vi "CheckRunGolden.vi"() -> ()   [LabVIEW 2012]
uses:
  <vilib>/addons/database/Auxilliary.llb/DB Tools Cursor Type.ctl
  <vilib>/addons/database/Connection.llb/DB Tools Open Connec (Path).vi
  <vilib>/addons/database/Connection.llb/Conn Execute.vi
  <vilib>/addons/database/Recordset.llb/Rec Destroy - Connection.vi
  <vilib>/addons/database/Recordset.llb/Rec Fetch Recordset Data (R).vi
  <vilib>/addons/database/_DB Variant To Data/Database Variant To Data.xnode
  <vilib>/addons/database/NI_Database_API.lvlib
panel:
  out "error out":errorcluster
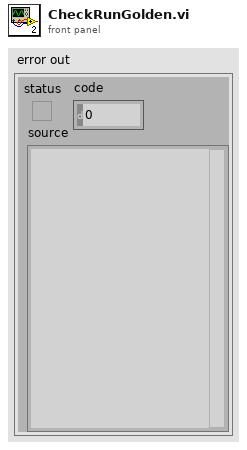
[diagram p1: front panel]
types:
  T1 = typedef "NI_Database_API.lvlib/DB Tools Cursor Type.ctl" = enum16{"forward-only", "keyset", "dynamic", "static"}
  T2 = typedef "NI_Database_API.lvlib/Conn ObjectReference.ctl" = refnum<k1>
  T3 = typedef "NI_Database_API.lvlib/Rec ObjectReference.ctl" = refnum<k1>
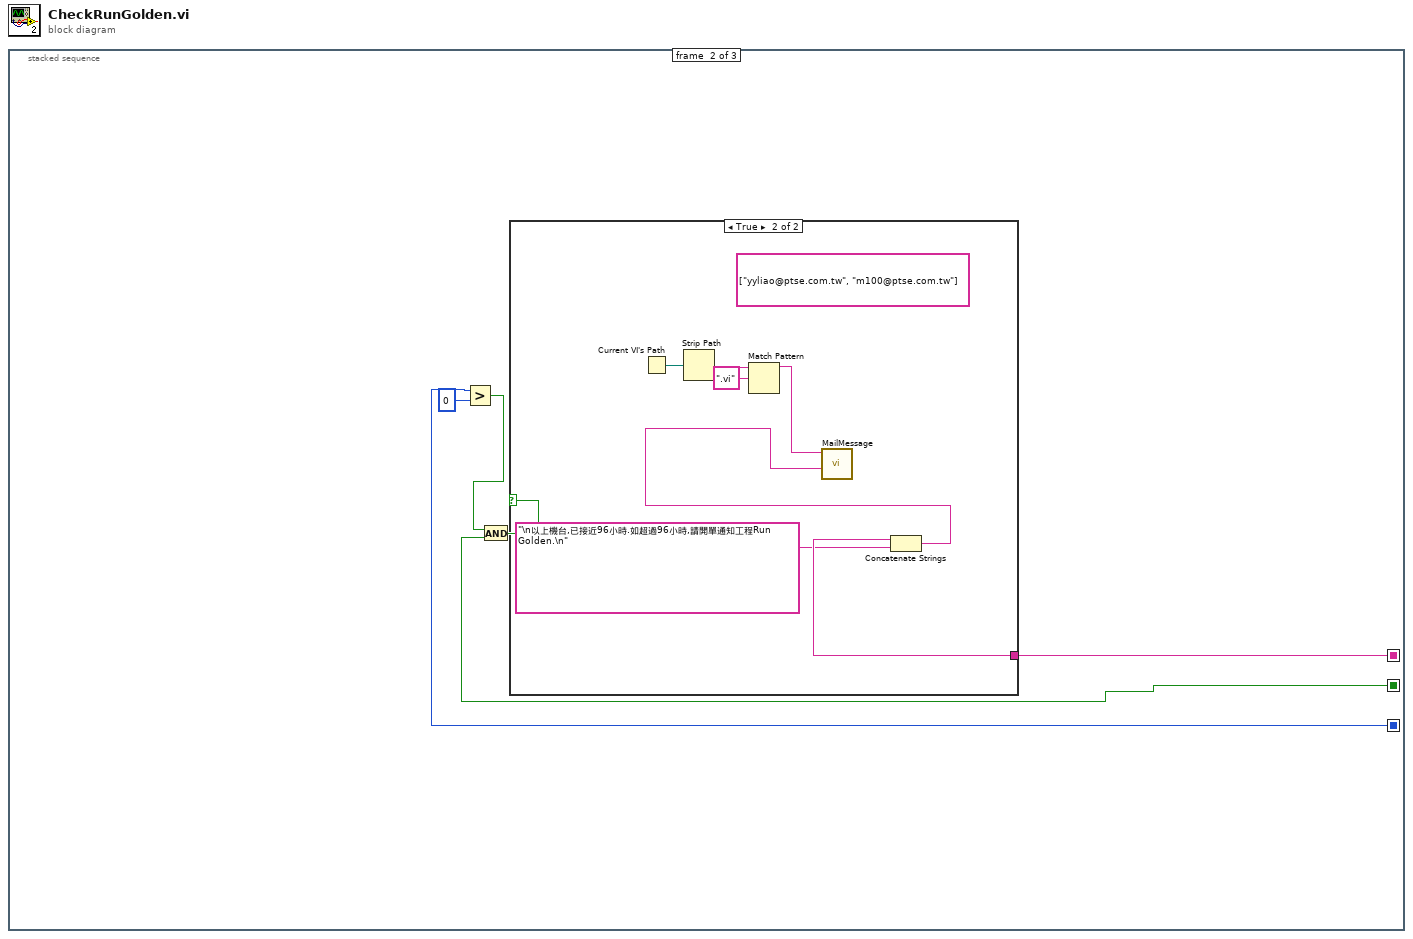
[diagram p0: block diagram]
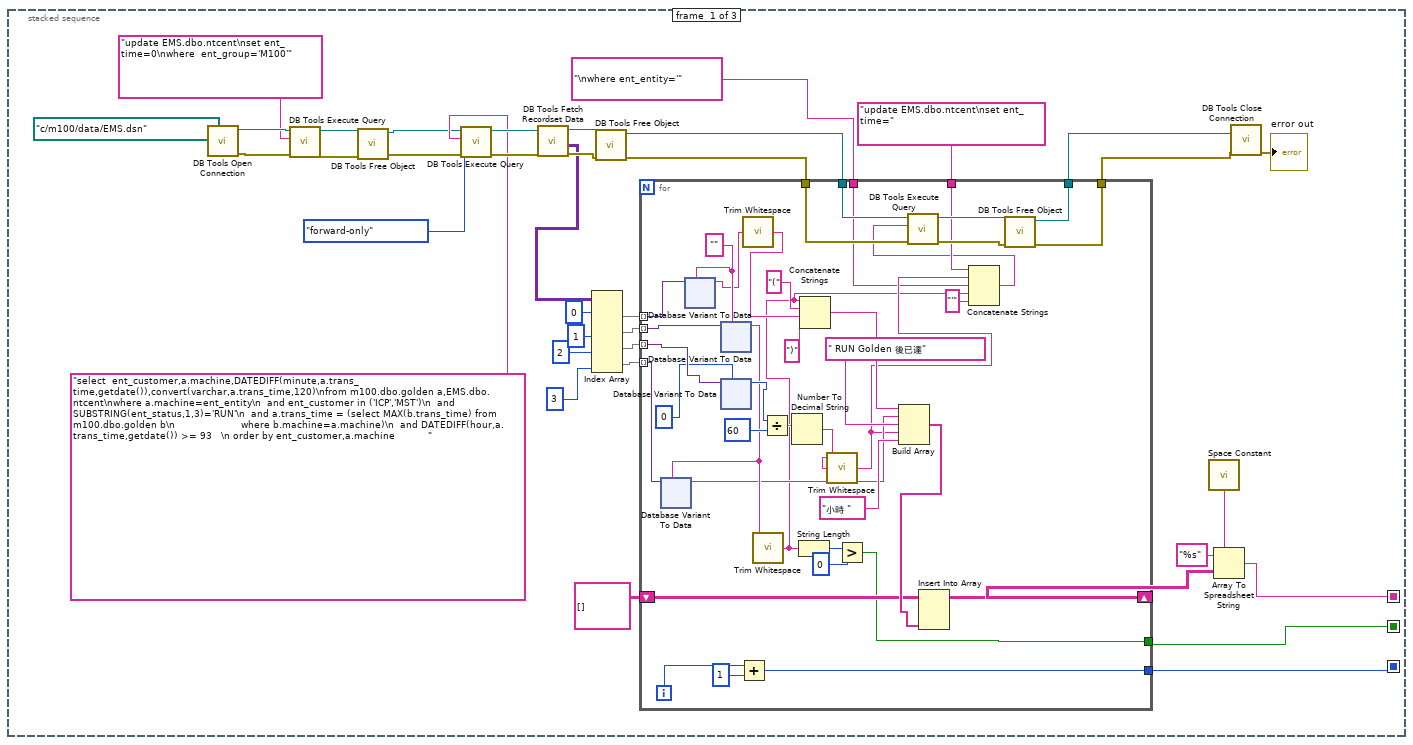
[diagram p2: hidden frame]
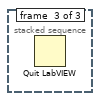
[diagram p4: hidden frame]
diagram:
  n1 = stacked-sequence {
    seq-local: [w24 _ _] -> [_ w211 _]
    seq-local: [w22 _ _] -> [_ w210 _]
    seq-local: [w21 _ _] -> [_ w206 _]
    frame #0 {
      n2 = call-poly <vilib>:"DB Tools Open Connection.vi"("connection information"=path "c:/m100/data/EMS.dsn") -> ("error out"=w2:errorcluster, "connection reference"=w8:T2)  [unwired: 7 in]
      n3 = call-poly <vilib>:"DB Tools Execute Query.vi"("error in (no error)"=w2, "SQL query"="update EMS.dbo.ntcent\nset ent_time=0\nwhere  ent_group='M100'", "connection reference"=w8) -> ("error out"=w3:errorcluster, "recordset reference"=w7:T3)  [unwired: 5 in]
      n4 = call-poly <vilib>:"DB Tools Free Object.vi"("error in (no error)"=w3, "recordset reference"=w7) -> ("error out"=w4:errorcluster, "connection reference"=w5:T2)  [unwired: 8 in]
      n5 = call-poly <vilib>:"DB Tools Execute Query.vi"("error in (no error)"=w4, "cursor type"=DB_Tools_Cursor_Type."forward-only", "SQL query"="select  ent_customer,a.machine,DATEDIFF(minute,a.trans_time,getdate()),convert(varchar,a.trans_time,120)\nfrom m100.dbo.golden a,EMS.dbo.ntcent\nwhere a.machine=ent_entity\n  and ent_customer in ('ICP','MST')\n  and SUBSTRING(ent_status,1,3)='RUN'\n  and a.trans_time = (select MAX(b.trans_time) from m100.dbo.golden b\n                      where b.machine=a.machine)\n  and DATEDIFF(hour,a.trans_time,getdate()) >= 93   \n order by ent_customer,a.machine           ", "connection reference"=w5) -> ("error out"=w35:errorcluster, "recordset reference"=w36:T3)  [unwired: 4 in]
      n6 = call-poly <vilib>:"DB Tools Fetch Recordset Data.vi"("error in (no error)"=w35, "recordset reference"=w36) -> ("error out"=w33:errorcluster, "recordset data"=w19:variant[][], "recordset reference out"=w34:T3)  [unwired: 3 in]
      n7 = Index Array(array=w19, index (col) #1=0 ("disabled index (col)"), index (col) #2=1 ("disabled index (col)"), index (col) #3=2 ("index (col)"), index (col) #4=3 ("index (col)")) -> (element #1=w17:variant[], element #2=w28:variant[], element #3=w27:variant[], element #4=w15:variant[])  [unwired: 4 in]
      n8 = call-poly <vilib>:"DB Tools Free Object.vi"("error in (no error)"=w33, "recordset reference"=w34) -> ("error out"=w12:errorcluster, "connection reference"=w14:T2)  [unwired: 8 in]
      n9 = for {
        tunnel: w28 -> [w77] mode=indexing
        tunnel: w27 -> [w76] mode=indexing
        shift-right: [w74] -> w25
        shift-left: string[][] [] -> [w73]
        tunnel: [w70] -> w22
        tunnel: [w67] -> w21
        tunnel: w17 -> [w59] mode=indexing
        tunnel: w15 -> [w53] mode=indexing
        tunnel: w14 -> [w49]
        tunnel: w12 -> [w48]
        tunnel: [w45] -> w13
        tunnel: [w44] -> w11
        tunnel: "update EMS.dbo.ntcent\nset ent_time=" -> [w43]
        tunnel: "\nwhere ent_entity='" ("string") -> [w41]
        i -> [w72]
        w58 = ""
        n10 = xnode "Database Variant To Data"("database variant"=w59, "type"=w58) -> ("data"=w55:string)  [unwired: 1 in, 1 out]
        n11 = xnode "Database Variant To Data"("database variant"=w77, "type"=w58) -> ("data"=w52:string)  [unwired: 1 in, 1 out]
        n12 = xnode "Database Variant To Data"("database variant"=w53, "type"=w52) -> ("data"=w50:string)  [unwired: 1 in, 1 out]
        n13 = xnode "Database Variant To Data"("database variant"=w76, "type"=0) -> ("data"=w64:i32)  [unwired: 1 in, 1 out]
        n14 = Add(x=w72, y=1) -> (x+y=w70:i32)
        n15 = call <vilib>:"Trim Whitespace.vi"("string"=w55) -> ("trimmed string"=w54:string)  [unwired: 1 in]
        n16 = call <vilib>:"Trim Whitespace.vi"("string"=w52) -> ("trimmed string"=w40:string)  [unwired: 1 in]
        n17 = Divide(x=w64, y=60) -> (x/y=w62:dbl)
        n18 = Number To Decimal String(number=w62) -> (decimal integer string=w60:string)  [unwired: 1 in]
        n19 = String Length(string=w40) -> (length=w69:i32)
        n20 = Concatenate Strings(w40, "(" ("string"), w54, ")" ("string")) -> (w51:string)
        n21 = call <vilib>:"Trim Whitespace.vi"("string"=w60) -> ("trimmed string"=w42:string)  [unwired: 1 in]
        n22 = Greater?(x=w69, y=0) -> (0:w67:bool)
        n23 = Build Array(w51, w50, " RUN Golden 後已達" ("element"), w42, "小時 " ("element")) -> (w75:string[])
        n24 = Insert Into Array(array=w73, new element=w75) -> (w74:string[][])  [unwired: 2 in]
        n25 = Concatenate Strings(w43, w42, w41, w40, "'" ("string")) -> (w38:string)
        n26 = call-poly <vilib>:"DB Tools Execute Query.vi"("error in (no error)"=w48, "SQL query"=w38, "connection reference"=w49) -> ("error out"=w46:errorcluster, "recordset reference"=w47:T3)  [unwired: 5 in]
        n27 = call-poly <vilib>:"DB Tools Free Object.vi"("error in (no error)"=w46, "recordset reference"=w47) -> ("error out"=w44:errorcluster, "connection reference"=w45:T2)  [unwired: 8 in]
      }
      n28 = call <vilib>:"Space Constant.vi"() -> ("String"=w23:string)
      n29 = Array To Spreadsheet String(delimiter (Tab)=w23, array=w25, 3:"%s" ("format string")) -> (spreadsheet string=w24:string)
      n30 = call <vilib>:"DB Tools Close Connection.vi"("error in (no error)"=w11, "connection reference"=w13) -> ("error out"=→"error out":errorcluster)  [unwired: 5 in]
    }
    frame #1 {
      n31 = Greater?(x=w210, y=0) -> (0:w208:bool)
      n32 = And(x=w208, y=w206) -> (x .and. y?=w207:bool)
      n33 = case shown="True" w207 {
        tunnel: w211 -> [_ w218]
        frame False {
        }
        frame True {
          (unwired) string[] ["yyliao@ptse.com.tw", "m100@ptse.com.tw"] ("recipients")
          n34 = Current VI's Path() -> (path=w216:path)
          n35 = Strip Path(path=w216) -> (name=w215:string)  [unwired: 1 out]
          n36 = Match Pattern(string=w215, regular expression=".vi") -> (before substring=w213:string)  [unwired: 1 in, 3 out]
          n37 = Concatenate Strings(w218, "\n以上機台,已接近96小時.如超過96小時,請開單通知工程Run Golden.\n" ("string")) -> (w212:string)
          n38 = call "MailMessage.vi"("message"=w212, "program"=w213) -> ()  [unwired: 10 in]
        }
      }
    }
    frame #2 {
      n39 = Quit LabVIEW() -> ()  [unwired: 1 in]
    }
  }
